vi "RNG(sus).vi"() -> ()   [LabVIEW 2016]
panel:
  out "Waveform Graph 4":dbl[](graph)
  out "Array 4":dbl[](array[numeric])
  out "Waveform Chart 4":dbl(graph)
  out "Waveform Graph 3":dbl[](graph)
  out "Array 3":dbl[](array[numeric])
  out "Waveform Chart 3":dbl(graph)
  out "Waveform Graph 2":dbl[](graph)
  out "Array 2":dbl[](array[numeric])
  out "Waveform Chart 2":dbl(graph)
  out "Waveform Graph":dbl[](graph)
  out "Waveform Chart":dbl(graph)
  out "Array":dbl[](array[numeric])
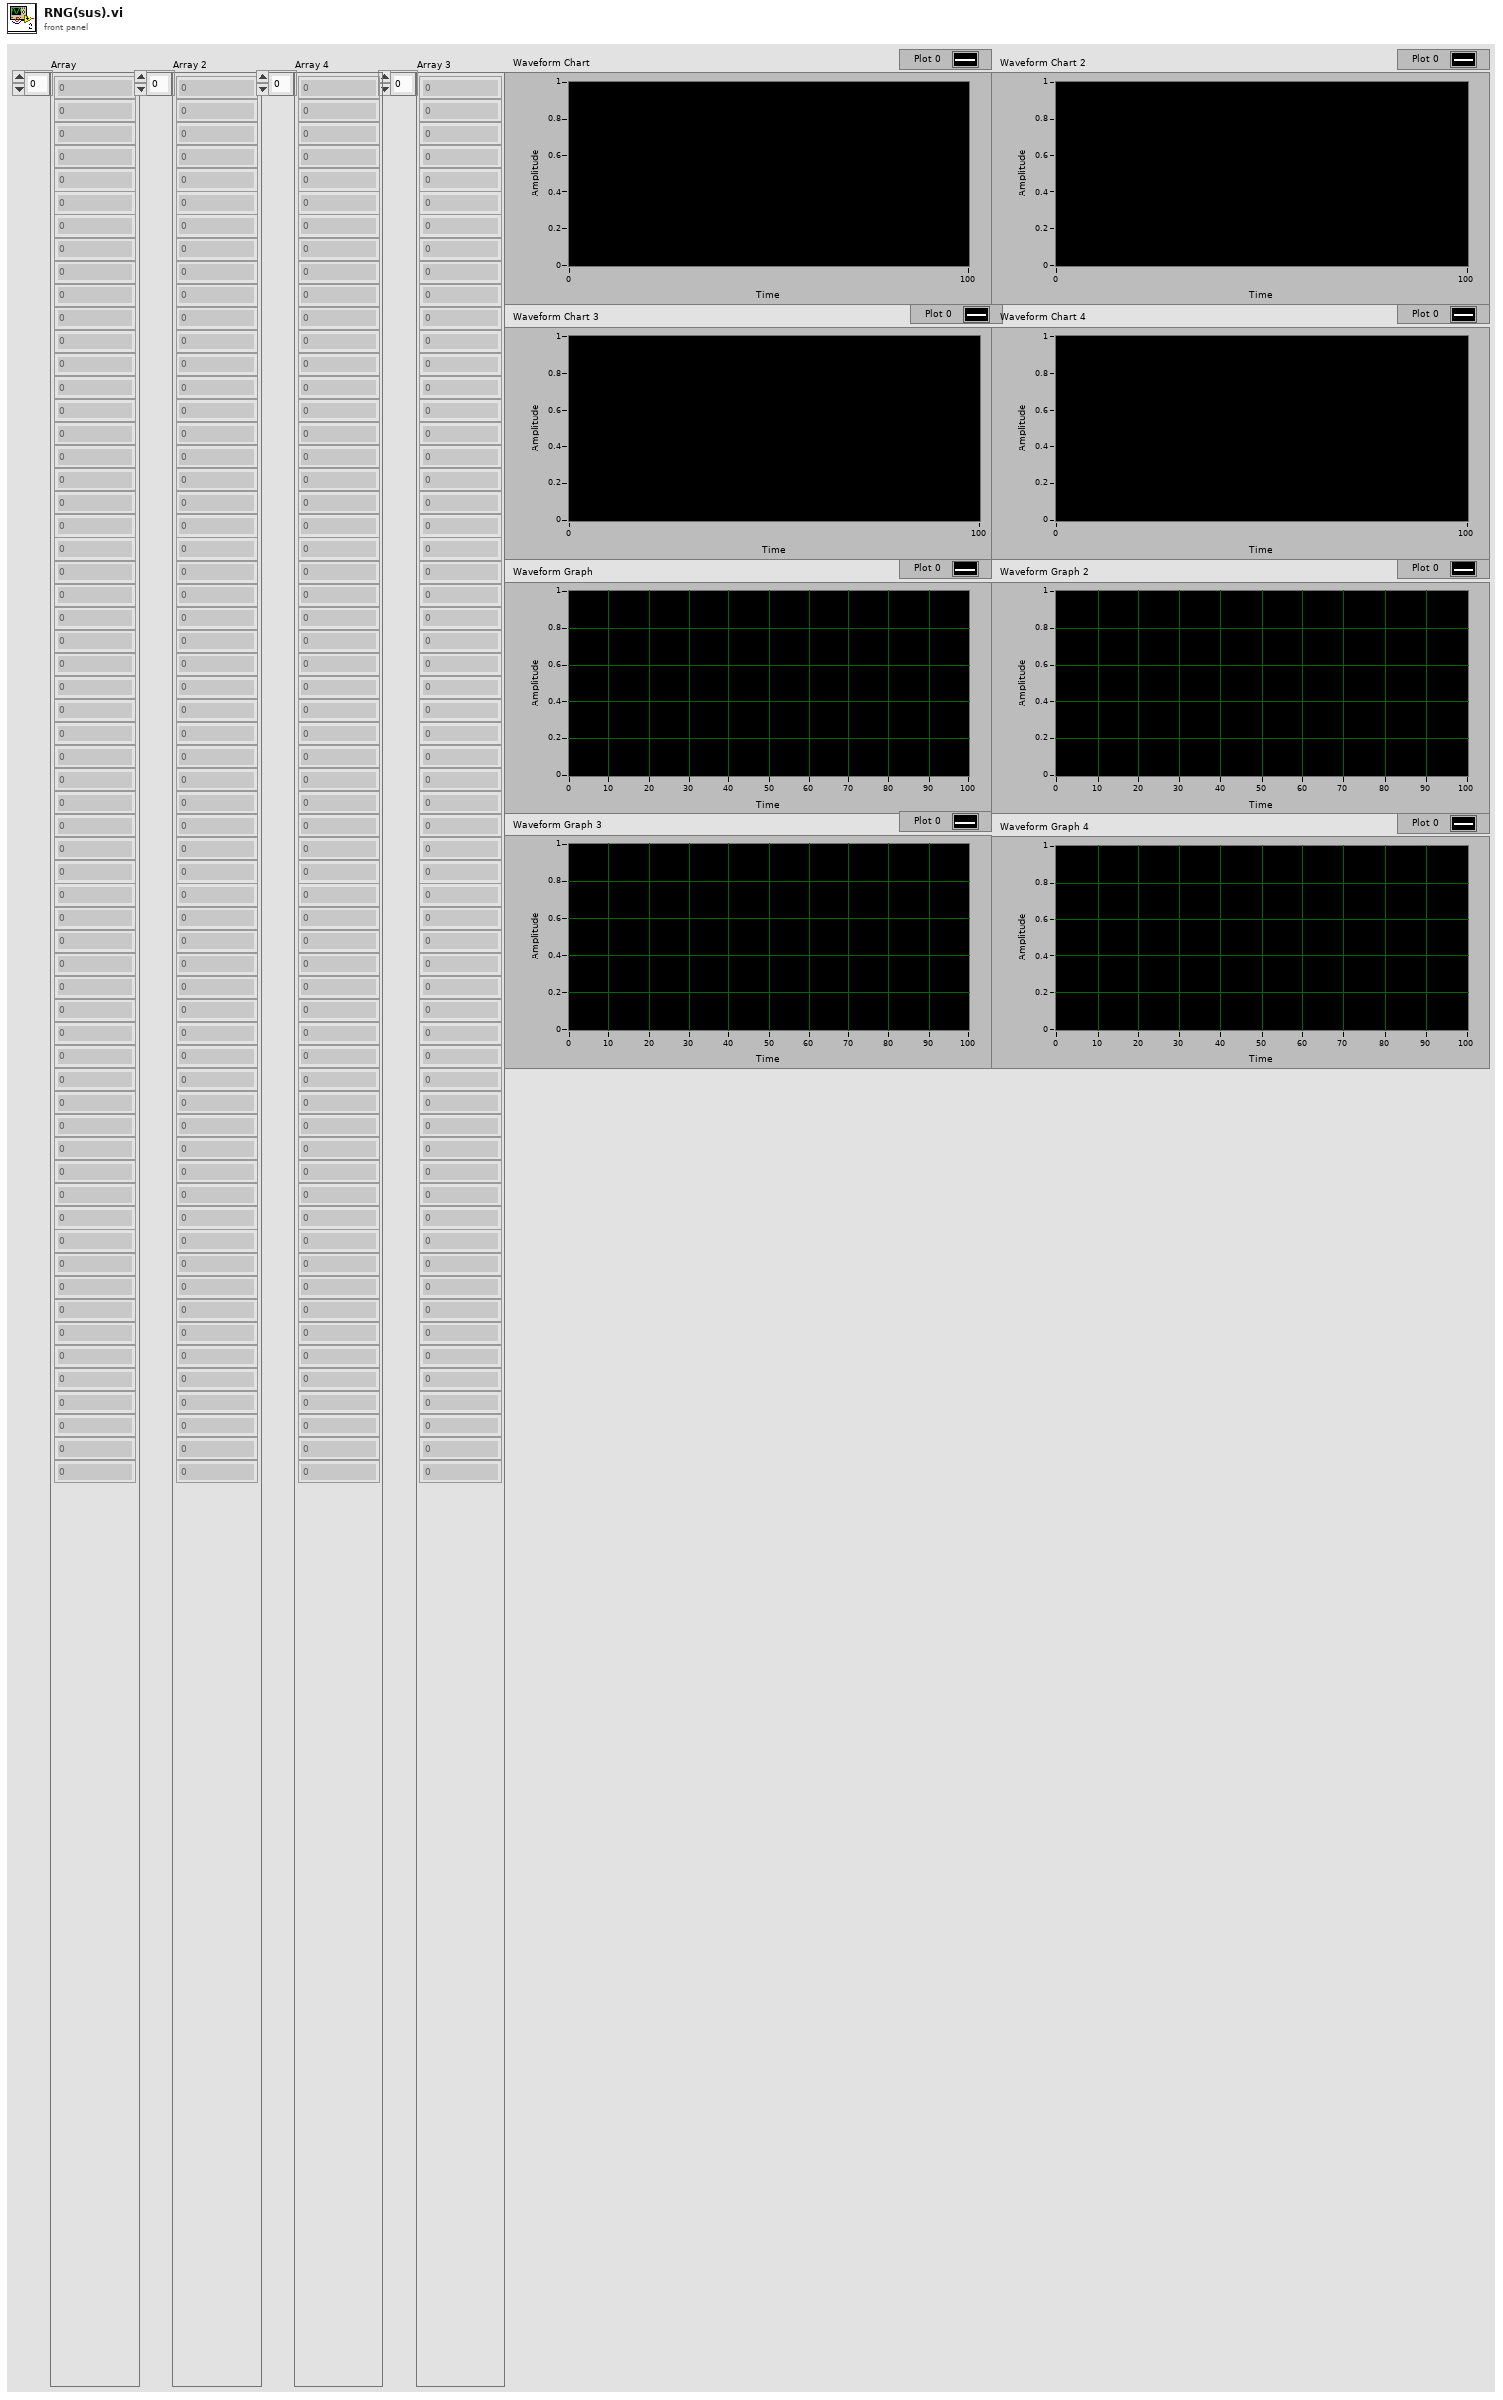
[diagram p1: front panel]
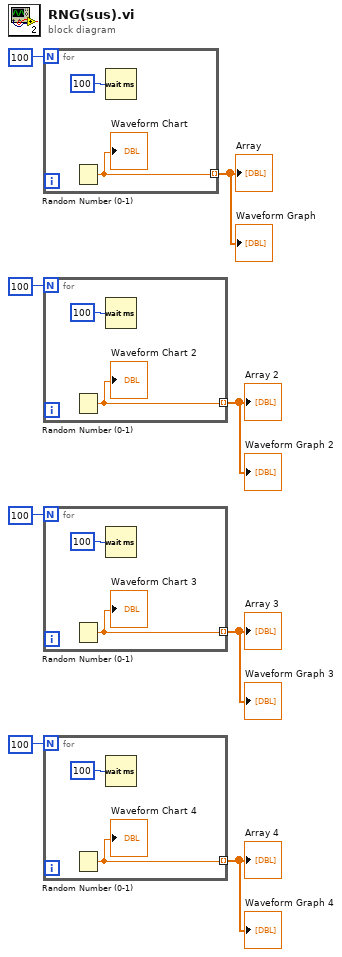
[diagram p0: block diagram]
diagram:
  n1 = for {
    N: 100 -> [_]
    tunnel: [w9] -> w6 mode=indexing
    n2 = Random Number (0-1)() -> (number: 0 to 1=w9:dbl)
    "Waveform Chart" <- w9
    n3 = Wait (ms)(milliseconds to wait=100) -> ()  [unwired: 1 out]
  }
  "Array" <- w6
  "Waveform Graph" <- w6
  n4 = for {
    N: 100 -> [_]
    tunnel: [w11] -> w5 mode=indexing
    n5 = Random Number (0-1)() -> (number: 0 to 1=w11:dbl)
    "Waveform Chart 2" <- w11
    n6 = Wait (ms)(milliseconds to wait=100) -> ()  [unwired: 1 out]
  }
  "Array 2" <- w5
  "Waveform Graph 2" <- w5
  n7 = for {
    N: 100 -> [_]
    tunnel: [w13] -> w2 mode=indexing
    n8 = Random Number (0-1)() -> (number: 0 to 1=w13:dbl)
    "Waveform Chart 3" <- w13
    n9 = Wait (ms)(milliseconds to wait=100) -> ()  [unwired: 1 out]
  }
  "Array 3" <- w2
  "Waveform Graph 3" <- w2
  n10 = for {
    N: 100 -> [_]
    tunnel: [w15] -> w1 mode=indexing
    n11 = Random Number (0-1)() -> (number: 0 to 1=w15:dbl)
    "Waveform Chart 4" <- w15
    n12 = Wait (ms)(milliseconds to wait=100) -> ()  [unwired: 1 out]
  }
  "Array 4" <- w1
  "Waveform Graph 4" <- w1
